vi "gentec-M-Link.Set Auto Range.vi"(0 "VISA resource In":refnum<visa-resource-name>, 2 "Auto Range":bool, 5 "error in (no error)":errorcluster) -> (11 "Data Read":string, 13 "Read Timeout":bool, 14 "VISA resource Out":refnum<visa-resource-name>, 17 "Success":bool, 19 "error out":errorcluster)   [LabVIEW 2014, in "gentec-M-Link - Driver.lvlib"]
doc: "Data to write: aut0 or aut1\n\nCommand only. Enables or Disables Auto Ranging: aut1 enables, aut0 disables Auto Range. Replies ok."
uses:
  gentec-M-Link - Driver.lvlib
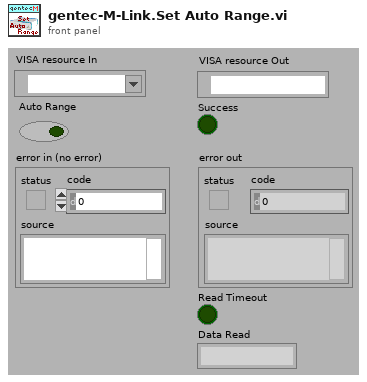
[diagram p1: front panel]
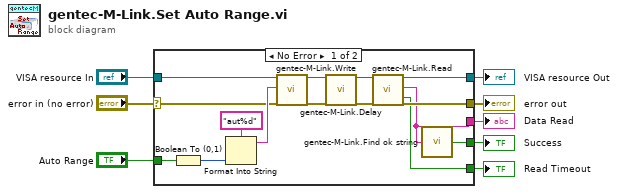
[diagram p0: block diagram]
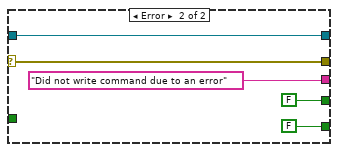
[diagram p2: hidden frame]
diagram:
  n1 = case shown="No Error" "error in (no error)" {
    selector: "error in (no error)" -> [w21 w28]
    tunnel: [w20 w28] -> w7
    tunnel: [w19 w27] -> w6
    tunnel: "VISA resource In" -> [w18 w27]
    tunnel: "Auto Range" -> [w17 _]
    tunnel: [w15 FALSE ("Found")] -> w3
    tunnel: [w13 "Did not write command due to an error" ("Data Read")] -> w2
    tunnel: [w12 FALSE ("Read Timeout")] -> w1
    frame No Error {
      n2 = Boolean To (0,1)(Boolean=w17) -> (0, 1=w14:i16)
      n3 = Format Into String(format string="aut%d", w14) -> (resulting string=w22:string)  [unwired: 2 in, 1 out]
      n4 = call "gentec-M-Link.Write.vi"("VISA resource (In)"=w18, "Data To Write"=w22, "error in (no error)"=w21) -> ("VISA resource (Out)"=w10:refnum<visa-resource-name>, "error out"=w16:errorcluster)  [unwired: 14 in, 1 out]
      n5 = call "gentec-M-Link.Delay.vi"("VISA resource In"=w10, "error in (no error)"=w16) -> ("VISA resource Out"=w9:refnum<visa-resource-name>, "error out"=w11:errorcluster)  [unwired: 16 in]
      n6 = call "gentec-M-Link.Read.vi"("VISA resource (In)"=w9, "error in (no error)"=w11) -> ("VISA resource (Out)"=w19:refnum<visa-resource-name>, "Data Read"=w13:string, "Read Timeout"=w12:bool, "error out"=w20:errorcluster)  [unwired: 13 in, 1 out]
      n7 = call "gentec-M-Link.Find ok string.vi"("string"=w13) -> ("Found"=w15:bool)
    }
    frame Error {
    }
  }
  "error out" <- w7
  "VISA resource Out" <- w6
  "Success" <- w3
  "Data Read" <- w2
  "Read Timeout" <- w1
